vi "cluster_v00.vi"() -> ()   [LabVIEW 2009]
uses:
  <vilib>/Platform/portaccess.llb/Out Port8.vi
panel:
  out "L6":bool=TRUE
  out "L4":bool=TRUE
  out "L5":bool
  out "L7":bool=TRUE
  out "L3":bool=TRUE
  out "L2":bool=TRUE
  out "L1":bool=TRUE
  in  "Selector":u8(knob) scale=0.0..9.0
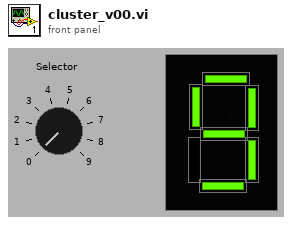
[diagram p1: front panel]
types:
  T1 = cluster{"Boolean array[0]":bool, "Boolean array[1]":bool, "Boolean array[2]":bool, "Boolean array[3]":bool, "Boolean array[4]":bool, "Boolean array[5]":bool, "Boolean array[6]":bool, "Boolean array[7]":bool}
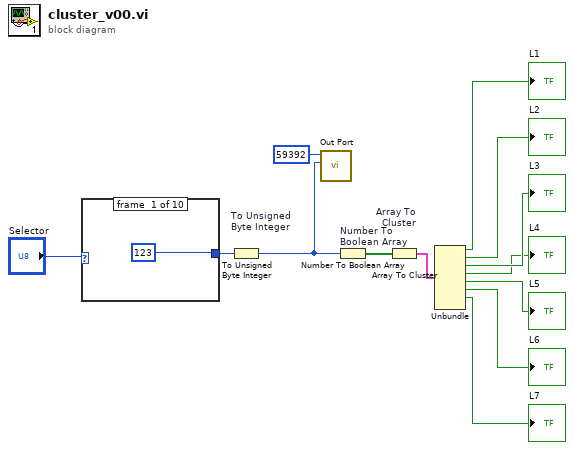
[diagram p0: block diagram]
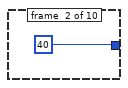
[diagram p2: hidden frame]
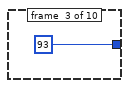
[diagram p3: hidden frame]
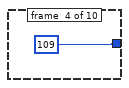
[diagram p4: hidden frame]
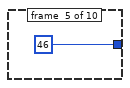
[diagram p5: hidden frame]
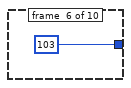
[diagram p6: hidden frame]
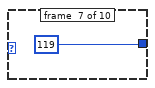
[diagram p7: hidden frame]
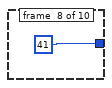
[diagram p8: hidden frame]
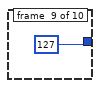
[diagram p9: hidden frame]
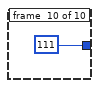
[diagram p10: hidden frame]
diagram:
  n1 = case shown="9" "Selector" {
    tunnel: [123 40 93 109 46 103 119 41 127 111] -> w12
    frame #0 {
    }
    frame #1 {
    }
    frame #2 {
    }
    frame #3 {
    }
    frame #4 {
    }
    frame #5 {
    }
    frame #6 {
    }
    frame #7 {
    }
    frame #8 {
    }
    frame #9 {
    }
  }
  n2 = To Unsigned Byte Integer "To Unsigned \nByte Integer"(number=w12) -> (unsigned 8bit integer=w1:u8)
  n3 = call-poly <vilib>:"Out Port.vi"("write value"=w1, "address"=59392) -> ()  [unwired: 7 in, 1 out]
  n4 = Number To Boolean Array "Number To \nBoolean Array"(number=w1) -> (Boolean array=w11:bool[])
  n5 = Array To Cluster "Array To \n  Cluster"(array=w11) -> (cluster=w10:T1)
  n6 = Unbundle "Unbundle"(w10) -> ("Boolean array[0]"=→"L1":bool, "Boolean array[1]"=→"L2":bool, "Boolean array[2]"=→"L3":bool, "Boolean array[3]"=→"L4":bool, "Boolean array[4]"=→"L5":bool, "Boolean array[5]"=→"L6":bool, "Boolean array[6]"=→"L7":bool)  [unwired: 1 out]
